vi "Read_File_AutoTest.vi"(8 "error in":errorcluster caption="entrée d'erreur (pas d'erreur)", 9 "Part Number PCBA":string(combo), 10 "Type Product":string(combo)="PCBA", 11 "file path":path) -> (0 "error out":errorcluster caption="sortie d'erreur", 1 "Instruments":T1(array[cluster]), 2 "Instrument List":string[](array[string]), 3 "Instr Class":refnum<class "Class Instrument (Default).lvclass">[](array[class]))   [LabVIEW 2020, in "Library Commun.lvlib"]
uses:
  Library Commun.lvlib
  Class/Instrument/Instrument (Default)/Class Instrument (Default).lvclass
  <vilib>/Utility/file.llb/Read Delimited Spreadsheet (string).vi
panel:
  # "This VI loads the Autotest CSV file and set the instrument object accordingly"
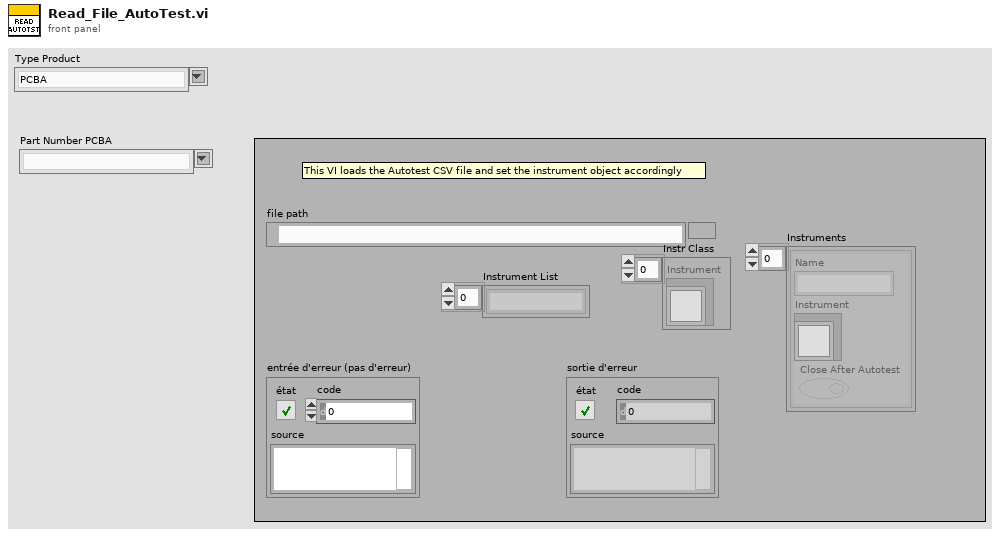
[diagram p1: front panel]
types:
  T1 = cluster{"Name":string, "Instrument":refnum<class "Class Instrument (Default).lvclass">, "Close After Autotest":bool}[]
  T2 = enum16{"Add Instr", "Remove Instr", "List Instr", "Get Instr Class", "Get Instr obj", "Save Insrt obj", "Modify Insrt obj", "Init"}
  T3 = cluster{"Name":string, "Instrument":refnum<class "Class Instrument (Default).lvclass">, "Close After Autotest":bool}
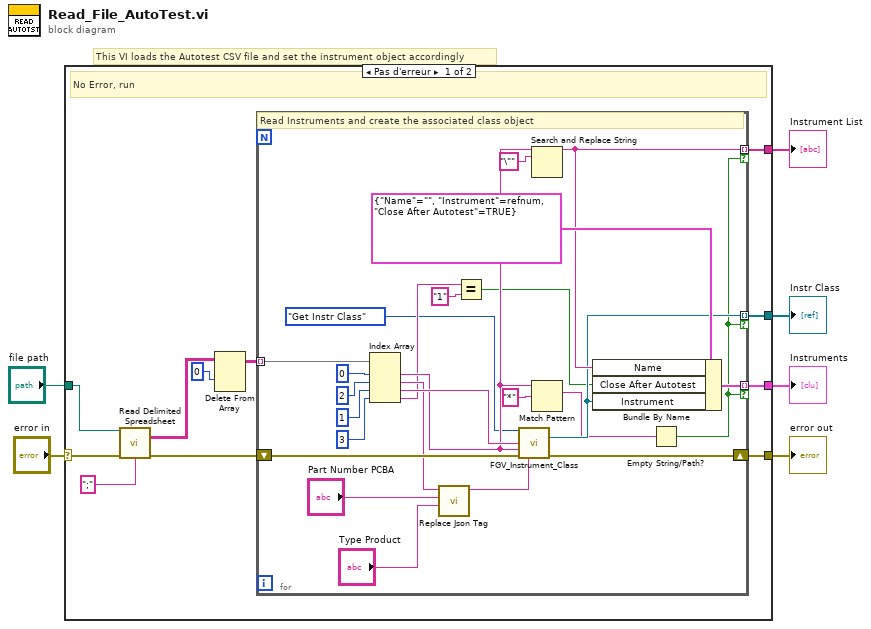
[diagram p0: block diagram]
diagram:
  # "This VI loads the Autotest CSV file and set the instrument object accordingly"
  n1 = case shown="Pas d'erreur" "error in" {
    selector: "error in" -> [w9 w43]
    tunnel: "file path" -> [w17 _]
    tunnel: [w11 w43] -> w5
    tunnel: [w10 _] -> w4
    tunnel: [w8 _] -> w2
    tunnel: [w7 _] -> w1
    frame No Error {
      # "No Error, run"
      n2 = call-poly <vilib>:"Read Delimited Spreadsheet.vi"("file path (dialog if empty)"=w17, "error in (no error)"=w9, "delimiter (\\t)"=";" ("delimiter (\\t)")) -> ("all rows"=w14:string[][], "error out"=w15:errorcluster)  [unwired: 7 in, 4 out]
      n3 = Delete From Array(array=w14, index (row)=0) -> (array with subset deleted=w13:string[][])  [unwired: 2 in, 1 out]
      n4 = for {
        tunnel: w13 -> [w39] mode=indexing
        shift-right: [w32] -> w11
        shift-left: w15 -> [w37]
        tunnel: [w31] -> w10 mode=indexing if=w27
        tunnel: [w34] -> w8 mode=indexing if=w27
        tunnel: [w33] -> w7 mode=indexing if=w27
        # "Read Instruments and create the associated class object"
        n5 = Index Array(array=w39, index #1=0 ("index"), index #2=2 ("index"), index #3=1 ("index"), index #4=3 ("indice")) -> (element #1=w30:string, element #2=w26:string, element #3=w36:string, element #4=w21:string)
        n6 = call "Replace Json Tag.vi"("Part Number PCBA"="Type Product", "Type Product"="Part Number PCBA", "Parameter (Json) en entrée"=w26) -> ("Parameter (Json) en sortie"=w25:string)  [unwired: 8 in]
        n7 = Equal?(x=w21, y="1") -> (x = y?=w19:bool)
        n8 = call "FGV_Instrument_Class.vi"("Action"=T2."Get Instr Class", "Instr class"=w36, "Instr name"=w30, "error in (no error)"=w37, "Parameter"=w25) -> ("Familly class Out"=w31:refnum<class "Class Instrument (Default).lvclass">, "error out"=w32:errorcluster)  [unwired: 8 in, 1 out]
        n9 = Search and Replace String(input string=w30, search string="\"") -> (result string=w34:string)  [unwired: 6 in, 3 out]
        n10 = Match Pattern(string=w30, regular expression="*" ("chaîne recherchée")) -> (match substring=w28:string)  [unwired: 1 in, 3 out]
        n11 = Bundle By Name(cluster=T3 {"Name"="", "Instrument"=refnum, "Close After Autotest"=TRUE} ("Cluster"), "Name"=w34, "Close After Autotest"=w19, "Instrument"=w31) -> (w33:T3)
        n12 = Empty String/Path?(string/path=w28) -> (empty?=w27:bool)
      }
    }
    frame Error {
      # "Error, do nothing"
    }
  }
  "error out" <- w5
  "Instr Class" <- w4
  "Instrument List" <- w2
  "Instruments" <- w1
